vi "Init Loop Data.vi"(11 "RemoteDataService in":refnum<class "RemoteDataService.lvclass">) -> (3 "Loop Data":T1 {"Published Groups"."Publish Address" format="%.0x"; "Published Groups"."Last Publish" format="%<%H:%M:%S%3u>T"})   [LabVIEW 2020, in "Vecto.lvlib" / "RemoteDataService.lvclass"]
uses:
  RemoteDataService.lvclass
  Loop Data.ctl
  SequenceCountService/SequenceCountService.lvclass
  Published Group.ctl
  Group/Group.lvclass
  RemoteDataService.lvclass/RemoteDataService.ctl
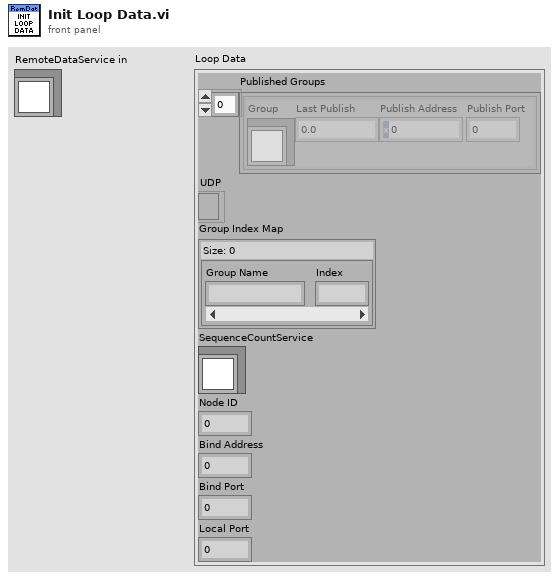
[diagram p1: front panel]
types:
  T1 = typedef "Vecto.lvlib/RemoteDataService.lvclass/Loop Data.ctl" = cluster{"Published Groups":T2[], "UDP":refnum<k16>, "Group Index Map":map{string, i32}, "SequenceCountService":refnum<class "SequenceCountService.lvclass">, "Node ID":u32, "Bind Address":u32, "Bind Port":u16, "Local Port":u16}
  T2 = typedef "Vecto.lvlib/RemoteDataService.lvclass/Published Group.ctl" = cluster{"Group":refnum<class "Group.lvclass">, "Last Publish":dbl, "Publish Address":u32, "Publish Port":u16}
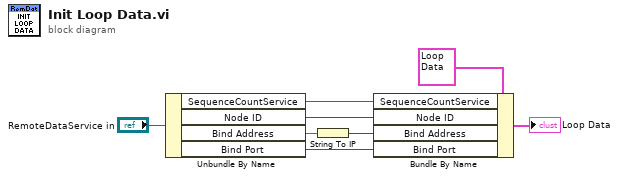
[diagram p0: block diagram]
diagram:
  n1 = Unbundle By Name("RemoteDataService in") -> ("SequenceCountService"=w5:refnum<class "SequenceCountService.lvclass">, "Node ID"=w4:u32, "Bind Address"=w3:string, "Bind Port"=w1:u16)
  n2 = String To IP(1:w3) -> (0:w2:u32)
  n3 = Bundle By Name(cluster=T1 {"Published Groups"=[], "UDP"=refnum, "Group Index Map"={}, "SequenceCountService"=refnum, "Node ID"=0, "Bind Address"=0, "Bind Port"=0, "Local Port"=0} ("Loop Data"), "SequenceCountService"=w5, "Node ID"=w4, "Bind Address"=w2, "Bind Port"=w1) -> (→"Loop Data":T1)
